vi "Recloser.vi"(6 "Current state":bool, 7 "Relay":bool, 8 "Counter In":dbl, 9 "Input array":fxp<+/-,26,5>[][](array[numeric]), 10 "Recloser Settings":T1, 11 "dt":dbl) -> (0 "Phase difference":dbl, 1 "frequency difference":dbl, 2 "magnitude difference":dbl, 3 "Recloser action":bool, 4 "Counter Out":dbl, 5 "Combined data for communication":dbl[](array[numeric]))   [LabVIEW 2016]
uses:
  <vilib>/Analysis/3filter.llb/Filter Passband Type.ctl
  <vilib>/Analysis/3filter.llb/Butterworth Filter (DBL).vi
  <vilib>/measure/matone.llb/Extract Single Tone Information N Chan.vi
  <vilib>/addons/Electrical Power/Basic/Measurement/RMS (N Channels).vi
  <vilib>/addons/Electrical Power/Basic/Measurement/Power (N Channels).vi
  <vilib>/addons/Electrical Power/Basic/NI_EP_Basic.lvlib
  <vilib>/measure/NI_MAPro.lvlib
  <vilib>/Analysis/NI_AALBase.lvlib
panel:
  in  "Waveform array":waveform(sgl)[](array[waveform])
  out "average phase diff":dbl
  out "RMS values VR":dbl[](array[numeric])
  out "RMS values VL":dbl[](array[numeric])
  out "VR array":waveform(sgl)[](array[waveform])
  out "VL array":waveform(sgl)[](array[waveform])
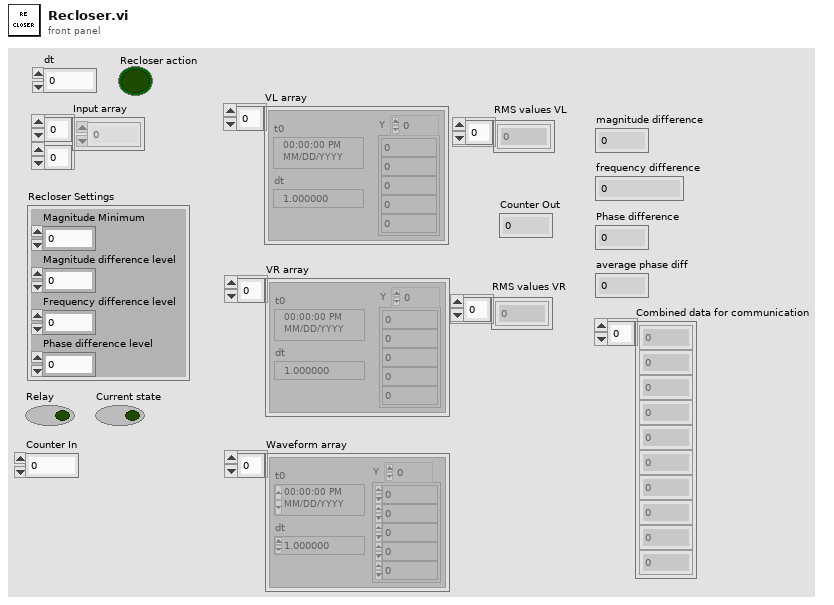
[diagram p1: front panel]
types:
  T1 = cluster{"Magnitude Minimum":dbl, "Magnitude difference level":dbl, "Frequency difference level":dbl, "Phase difference level":dbl}
  T2 = typedef "NI_AALBase.lvlib/Filter Passband Type.ctl" = enum32{"Lowpass", "Highpass", "Bandpass", "Bandstop"}
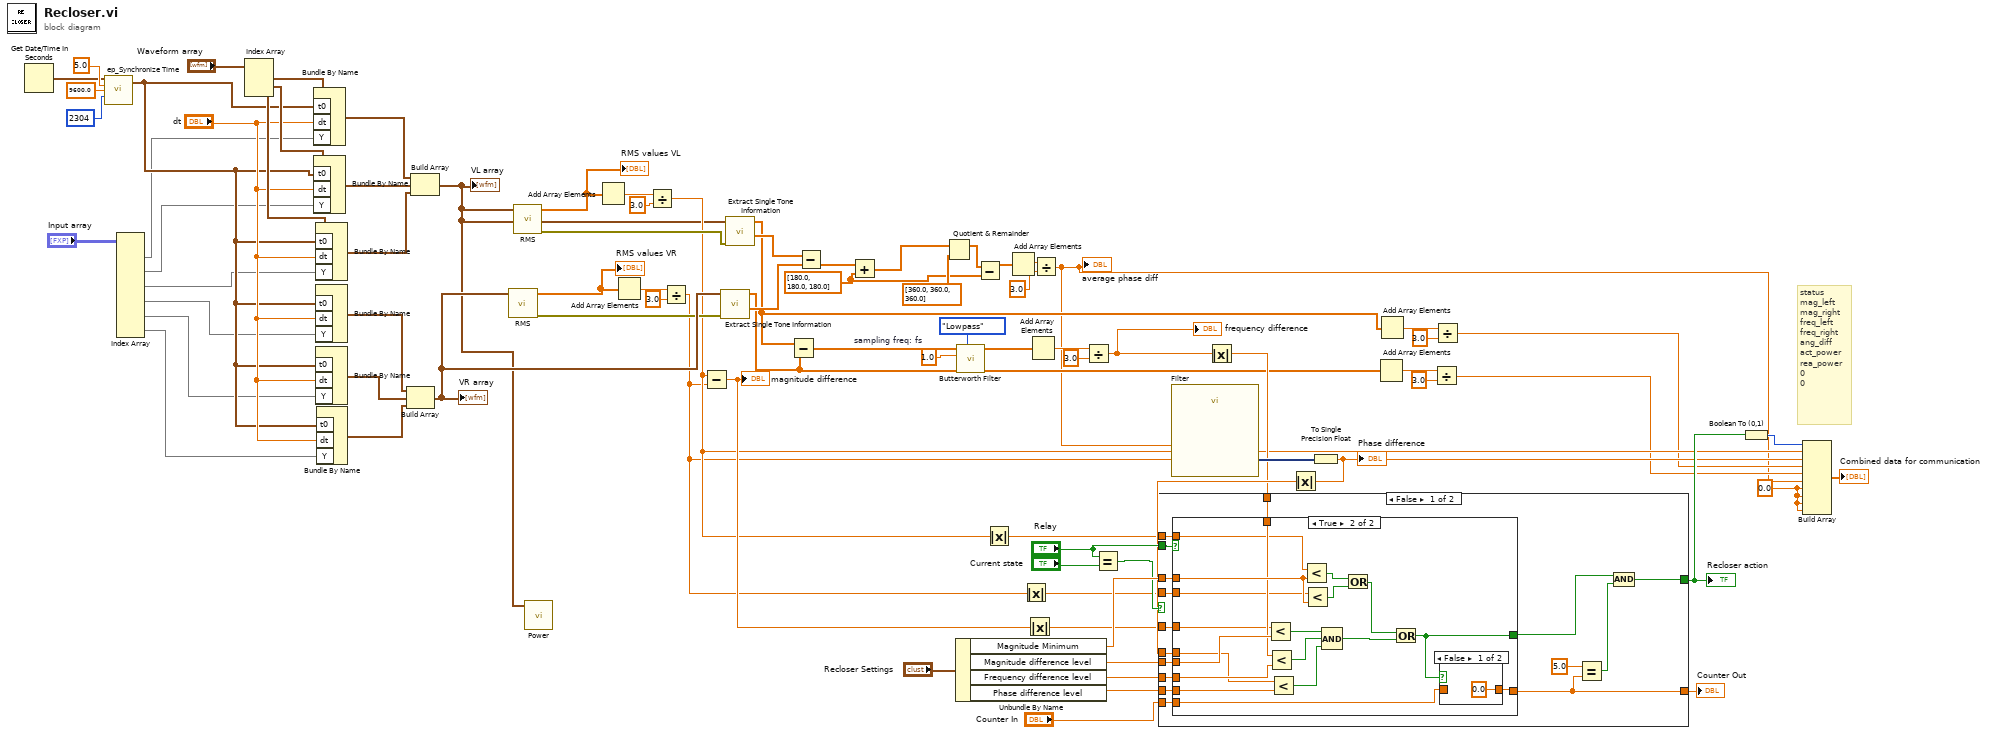
[diagram p0: block diagram]
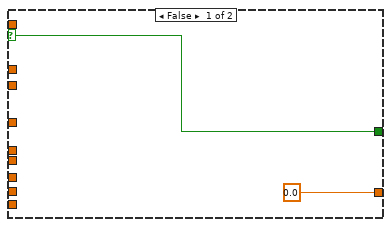
[diagram p2: hidden frame]
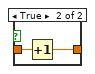
[diagram p3: hidden frame]
diagram:
  w2 = 0.0 ("element")
  w35 = 1.0  # sampling freq: fs
  w34 = dbl[] [180.0, 180.0, 180.0] ("y")
  # "status\nmag_left\nmag_right\nfreq_left\nfreq_right\nang_diff\nact_power\nrea_power\n0\n0"
  n1 = Get Date/Time In Seconds() -> (seconds since 1Jan1904=w71:timestamp)
  n2 = call <vilib>:"ep_Synchronize Time.vi"("RT controler time in"=w71, "maximum time difference (sec)"=5.0, "sampling rate (Hz)"=9600.0, "basic calc. interval (samples)"=2304) -> ("RT controler time out"=w70:timestamp)  [unwired: 11 in]
  n3 = Index Array(array="Input array") -> (element #1=w42:fxp<+/-,26,5>[], element #2=w41:fxp<+/-,26,5>[], element #3=w40:fxp<+/-,26,5>[], element #4=w39:fxp<+/-,26,5>[], element #5=w38:fxp<+/-,26,5>[], element #6=w37:fxp<+/-,26,5>[])  [unwired: 12 in]
  n4 = Index Array(array="Waveform array") -> (element #1=w83:waveform(sgl), element #2=w82:waveform(sgl), element #3=w81:waveform(sgl))  [unwired: 3 in]
  n5 = Bundle By Name(cluster=w83, "t0"=w70, "dt"="dt", "Y"=w42) -> (w78:waveform(sgl))
  n6 = Bundle By Name(cluster=w82, "t0"=w70, "dt"="dt", "Y"=w41) -> (w77:waveform(sgl))
  n7 = Bundle By Name(cluster=w81, "t0"=w70, "dt"="dt", "Y"=w40) -> (w76:waveform(sgl))
  n8 = Bundle By Name("t0"=w70, "dt"="dt", "Y"=w39) -> (w74:waveform(sgl))  [unwired: 1 in]
  n9 = Bundle By Name("t0"=w70, "dt"="dt", "Y"=w38) -> (w73:waveform(sgl))  [unwired: 1 in]
  n10 = Bundle By Name("t0"=w70, "dt"="dt", "Y"=w37) -> (w72:waveform(sgl))  [unwired: 1 in]
  n11 = Build Array(w74, w73, w72) -> (w48:waveform(sgl)[])
  "VR array" <- w48
  n12 = Build Array(w78, w77, w76) -> (w4:waveform(sgl)[])
  "VL array" <- w4
  n13 = call-poly <vilib>:"RMS.vi"("waveforms"=w48) -> ("error out"=w45:errorcluster, "RMS values"=w60:dbl[])  [unwired: 9 in]
  "RMS values VR" <- w60
  n14 = call-poly <vilib>:"RMS.vi"("waveforms"=w4) -> ("error out"=w68:errorcluster, "RMS values"=w63:dbl[])  [unwired: 9 in]
  "RMS values VL" <- w63
  n15 = call-poly <vilib>:"Power.vi"("voltage waveforms"=w4) -> ()  [unwired: 9 in, 2 out]
  n16 = Add Array Elements(numeric array=w63) -> (sum=w62:dbl)
  n17 = Add Array Elements(numeric array=w60) -> (sum=w65:dbl)
  n18 = Divide(x=w62, y=3.0) -> (x/y=w14:dbl)
  n19 = Divide(x=w65, y=3.0) -> (x/y=w13:dbl)
  n20 = Subtract(x=w14, y=w13) -> (x-y=w27:dbl)
  "magnitude difference" <- w27
  n21 = call-poly <vilib>:"Extract Single Tone Information.vi"("error in (no error)"=w45, "time signals in"=w48) -> ("detected phases (deg)"=w66:dbl[], "detected frequencies"=w5:dbl[])  [unwired: 4 in, 4 out]
  n22 = call-poly <vilib>:"Extract Single Tone Information.vi"("error in (no error)"=w68, "time signals in"=w4) -> ("detected phases (deg)"=w69:dbl[], "detected frequencies"=w8:dbl[])  [unwired: 4 in, 4 out]
  n23 = Subtract(x=w8, y=w5) -> (x-y=w47:dbl[])
  n24 = Subtract(x=w69, y=w66) -> (x-y=w67:dbl[])
  n25 = Add(x=w67, y=w34) -> (x+y=w46:dbl[])
  n26 = Quotient & Remainder(x=w46, y=dbl[] [360.0, 360.0, 360.0]) -> (x-y*floor(x/y)=w55:dbl[])  [unwired: 1 out]
  n27 = Unbundle By Name("Recloser Settings") -> ("Magnitude Minimum"=w33:dbl, "Magnitude difference level"=w32:dbl, "Frequency difference level"=w31:dbl, "Phase difference level"=w30:dbl)
  n28 = call-poly <vilib>:"Butterworth Filter.vi"("filter type"=Filter_Passband_Type."Lowpass", "sampling freq: fs"=w35, "X"=w47) -> ("Filtered X"=w53:dbl[])  [unwired: 5 in, 1 out]
  n29 = Subtract(x=w55, y=w34) -> (x-y=w54:dbl[])
  n30 = Absolute Value(x=w14) -> (abs(x)=w18:dbl)
  n31 = Add Array Elements(numeric array=w54) -> (sum=w58:dbl)
  n32 = Absolute Value(x=w13) -> (abs(x)=w19:dbl)
  n33 = Absolute Value(x=w27) -> (abs(x)=w20:dbl)
  n34 = Add Array Elements(numeric array=w53) -> (sum=w51:dbl)
  n35 = Divide(x=w58, y=3.0 ("x")) -> (x/y=w3:dbl)
  "average phase diff" <- w3
  n36 = Divide(x=w51, y=3.0) -> (x/y=w28:dbl)
  "frequency difference" <- w28
  n37 = Equal?(x="Relay", y="Current state") -> (x = y?=w24:bool)
  n38 = call "Filter"("Signal"=w3) -> ("Filtered Signal"=w52:dynamicdata)  [unwired: 9 in, 1 out]
  n39 = Absolute Value(x=w28) -> (abs(x)=w17:dbl)
  n40 = To Single Precision Float(number=w52) -> (single precision float=w29:sgl)
  "Phase difference" <- w29
  n41 = Absolute Value(x=w29) -> (abs(x)=w21:sgl)
  n42 = case shown="False" w24 {
    tunnel: [w96 _] -> w25
    tunnel: [w97 w124] -> w15
    tunnel: w33 -> [w94 _]
    tunnel: w32 -> [w93 _]
    tunnel: w31 -> [w92 _]
    tunnel: w30 -> [w91 _]
    tunnel: w21 -> [w90 _]
    tunnel: w17 -> [w89 _]
    tunnel: w20 -> [w88 _]
    tunnel: "Relay" -> [w87 w124]
    tunnel: "Counter In" -> [w86 _]
    tunnel: w18 -> [w85 _]
    tunnel: w19 -> [w84 _]
    frame False {
      n43 = case shown="True" w87 {
        selector: w87 -> [w101 _]
        tunnel: [w101 w112] -> w95
        tunnel: [0.0 w113] -> w96
        tunnel: w94 -> [_ w111]
        tunnel: w93 -> [_ w110]
        tunnel: w92 -> [_ w109]
        tunnel: w91 -> [_ w108]
        tunnel: w90 -> [_ w107]
        tunnel: w89 -> [_ w106]
        tunnel: w88 -> [_ w105]
        tunnel: w86 -> [_ w104]
        tunnel: w85 -> [_ w103]
        tunnel: w84 -> [_ w102]
        frame False {
        }
        frame True {
          n44 = Less?(x=w105, y=w110) -> (x < y?=w115:bool)
          n45 = Less?(x=w106, y=w109) -> (x < y?=w118:bool)
          n46 = Less?(x=w107, y=w108) -> (x < y?=w117:bool)
          n47 = Less?(x=w103, y=w111) -> (x < y?=w120:bool)
          n48 = Less?(x=w102, y=w111) -> (x < y?=w119:bool)
          n49 = Compound Arithmetic op=AND(w115, w118, w117) -> (w116:bool)
          n50 = Or(x=w120, y=w119) -> (x .or. y?=w114:bool)
          n51 = Or(x=w114, y=w116) -> (x .or. y?=w112:bool)
          n52 = case shown="False" w112 {
            tunnel: [0.0 w123] -> w113
            tunnel: w104 -> [_ w122]
            frame False {
            }
            frame True {
              n53 = Increment(x=w122) -> (x+1=w123:dbl)
            }
          }
        }
      }
      n54 = Equal?(x=5.0, y=w96) -> (x = y?=w98:bool)
      n55 = And(x=w95, y=w98) -> (x .and. y?=w97:bool)
    }
    frame True {
    }
  }
  "Recloser action" <- w15
  "Counter Out" <- w25
  n56 = Add Array Elements(numeric array=w5) -> (sum=w10:dbl)
  n57 = Add Array Elements(numeric array=w8) -> (sum=w11:dbl)
  n58 = Divide(x=w10, y=3.0) -> (x/y=w6:dbl)
  n59 = Divide(x=w11, y=3.0) -> (x/y=w7:dbl)
  n60 = Boolean To (0,1)(Boolean=w15) -> (0, 1=w16:i16)
  n61 = Build Array(w16, w14, w13, w7, w6, w3, w2, w2, w2, w2) -> (→"Combined data for communication":dbl[])
